vi "Setup.vi"(8 "error in (no error)":errorcluster, 11 "LUnit Test Case In":refnum<class "Setup Error Test Dummy.lvclass">) -> (0 "error out":errorcluster, 3 "LUnit Test Case Out":refnum<class "Setup Error Test Dummy.lvclass">)   [LabVIEW 2020, in "Setup Error Test Dummy.lvclass"]
doc: "Setup method called by the testing framework before each test method is called."
uses:
  Setup Error Test Dummy.lvclass
  Setup Error Test Dummy.lvclass/Setup Error Test Dummy.ctl
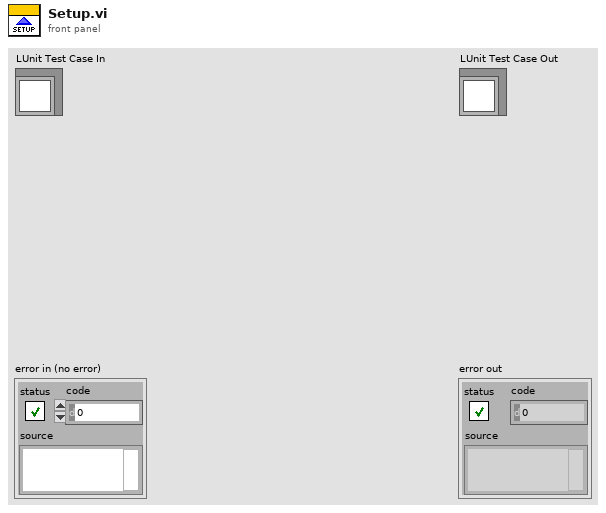
[diagram p1: front panel]
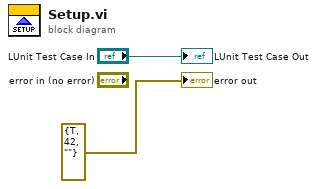
[diagram p0: block diagram]
diagram:
  "error out" <- errorcluster {"status"=TRUE, "code"=42, "source"=""} ("error out")
  "LUnit Test Case Out" <- "LUnit Test Case In"
